vi "Set Output.vi"(8 "error in":errorcluster, 9 "State":bool, 10 "portBit":i32=-1, 11 "task in":i32) -> (0 "error out":errorcluster, 3 "task out":i32)   [LabVIEW 2025, in "DIO.lvlib"]
uses:
  DIO.lvlib
  <userlib>/DAQNavi Polymorphic VI/write/DAQNavi Write (Digital U8 1Chan 1Samp).vi
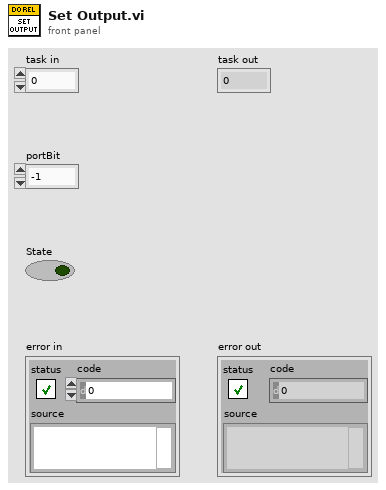
[diagram p1: front panel]
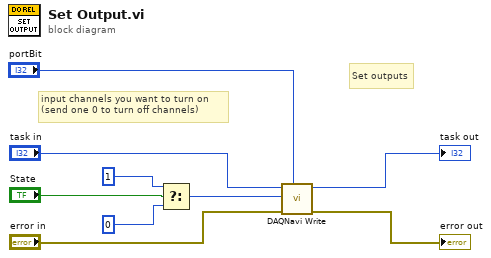
[diagram p0: block diagram]
diagram:
  # "Set outputs"
  # "input channels you want to turn on\n(send one 0 to turn off channels)"
  n1 = Select(t=u8 1 ("data"), s="State", f=u8 0 ("data")) -> (s? t:f=w2:u8)
  n2 = call-poly <userlib>:"DAQNavi Write.vi"("portBit"="portBit", "error in (no error)"="error in", "data"=w2, "task in"="task in") -> ("error out"=→"error out":errorcluster, "task out"=→"task out":i32)  [unwired: 1 in, 5 out]
